vi "temperature_unit_converter.vi"(1 "Output Unit [K]":string(combo)="K", 2 "Input":dbl format="%#_13g", 3 "Input Unit  [C]":string(combo)="C") -> (0 "Output":dbl)   [LabVIEW 2017, in "sensor_translation.lvlib"]
uses:
  sensor_translation.lvlib
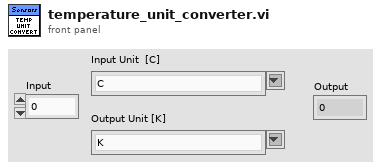
[diagram p1: front panel]
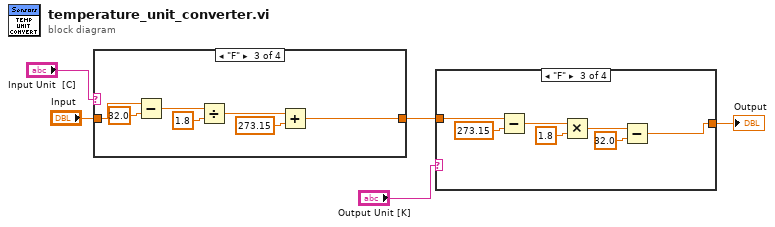
[diagram p0: block diagram]
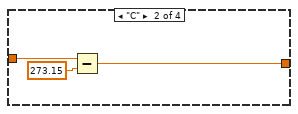
[diagram p3: hidden frame]
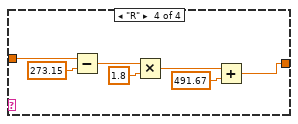
[diagram p4: hidden frame]
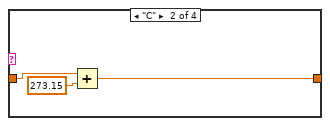
[diagram p6: hidden frame]
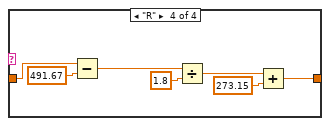
[diagram p7: hidden frame]
diagram:
  n1 = case shown="\"F\"" "Input Unit  [C]" {
    tunnel: "Input" -> [w6 w9 w14 w23]
    tunnel: [w6 w7 w15 w17] -> w2
    frame "K", Default {
      # "First convert to Kelvin"
    }
    frame "C" {
      n2 = Add(x=w9, y=273.15) -> (x+y=w7:dbl)
    }
    frame "F" {
      n3 = Subtract(x=w14, y=32.0) -> (x-y=w12:dbl)
      n4 = Divide(x=w12, y=1.8) -> (x/y=w10:dbl)
      n5 = Add(x=w10, y=273.15) -> (x+y=w15:dbl)
    }
    frame "R" {
      n6 = Subtract(x=w23, y=491.67) -> (x-y=w21:dbl)
      n7 = Divide(x=w21, y=1.8) -> (x/y=w19:dbl)
      n8 = Add(x=w19, y=273.15) -> (x+y=w17:dbl)
    }
  }
  n9 = case shown="\"F\"" "Output Unit [K]" {
    tunnel: w2 -> [w24 w25 w34 w41]
    tunnel: [w24 w26 w28 w35] -> w1
    frame "K", Default {
      # "First convert to Kelvin"
    }
    frame "C" {
      n10 = Subtract(x=w25, y=273.15) -> (x-y=w26:dbl)
    }
    frame "F" {
      n11 = Subtract(x=w34, y=273.15) -> (x-y=w32:dbl)
      n12 = Multiply(x=w32, y=1.8) -> (x*y=w30:dbl)
      n13 = Subtract(x=w30, y=32.0) -> (x-y=w28:dbl)
    }
    frame "R" {
      n14 = Subtract(x=w41, y=273.15) -> (x-y=w38:dbl)
      n15 = Multiply(x=w38, y=1.8) -> (x*y=w37:dbl)
      n16 = Add(x=w37, y=491.67) -> (x+y=w35:dbl)
    }
  }
  "Output" <- w1
